vi "MAIN_test.vi"() -> ()   [LabVIEW 2023]
uses:
  <vilib>/Utility/file.llb/Write Delimited Spreadsheet (string).vi
  <vilib>/Utility/file.llb/Write Delimited Spreadsheet (I64).vi
  BT-Android_AE_library/BT-Android_interface.lvlib
  <resource>/objmgr/ni.dex.rc
panel:
  out "数组 4":i32[](array[numeric])
  out "数组 3":i32[](array[numeric])
  in  "?":enum32{"other test", "test 2"}(tab)
  out "End Character?":bool
  out "send timeout":bool=TRUE
  out "?":bool=TRUE
  in  "Send":bool
  in  "Data Send":string
  in  "Close Com":bool
  in  "timeout (10sec)":u32=10000
  out "status":bool
  out "code":i32
  out "source":string
  in  "temp varible":u16=4660 format="%x"
  out "single":u16(graph)
  in  "?":enum32{"初始化", "dynamic", "测试"}(tab)
  in  "local baud rate":u32=1000000
  in  "Select COM before run":refnum<visa-resource-name>="COM5"
  in  "Channels（包括检验）":i32=33
  in  "receive query frequency(ms)":i32=1
  in  "VISA size set":i32=10000
  in  "error queue size":i32=-1
  in  "receive file path (dialog if empty)":path=path "D:/Proj-labview/蓝牙无线采集/wireless-console/sd_data"
  in  "开始采集":bool
  in  "结束采集":bool
  out "data stream ele":i32
  out "VISA bytes now":i32
  in  "VISA bytes max":i32
  out "本次采样用时s":dbl format="%.2f"
  out "display array":u16[](array[numeric])
  out "接收字符串":string
  in  "采集选项":u16(ring) items=["上位机采集", "sd卡采集"]
  out "开始时间点":string="时间点字符串"
  in  "Receive":bool=TRUE
  out "data16 stream ele":i32
  in  "data16 save max":i32
  in  "data存盘":bool
  out "采样率PS":dbl format="%#_13g"
  out "Average Error Ratio":dbl format="%#.4f"
  in  "Right cycle":u64
  in  "Error cycle":i32
  in  "更新采样信息":bool=TRUE
  in  "error存盘":bool
  in  "mod":u8
  in  "清缓存":bool
  in  "data max ele":i32
  out "本次采样开始时间ms":u64
  in  "固定字符测试":bool
  out "时间打点":u64
  out "right cycle打点":u64
  out "35通道波形":u16[][](graph)
  # "通用设置："
  # "蓝牙设置："
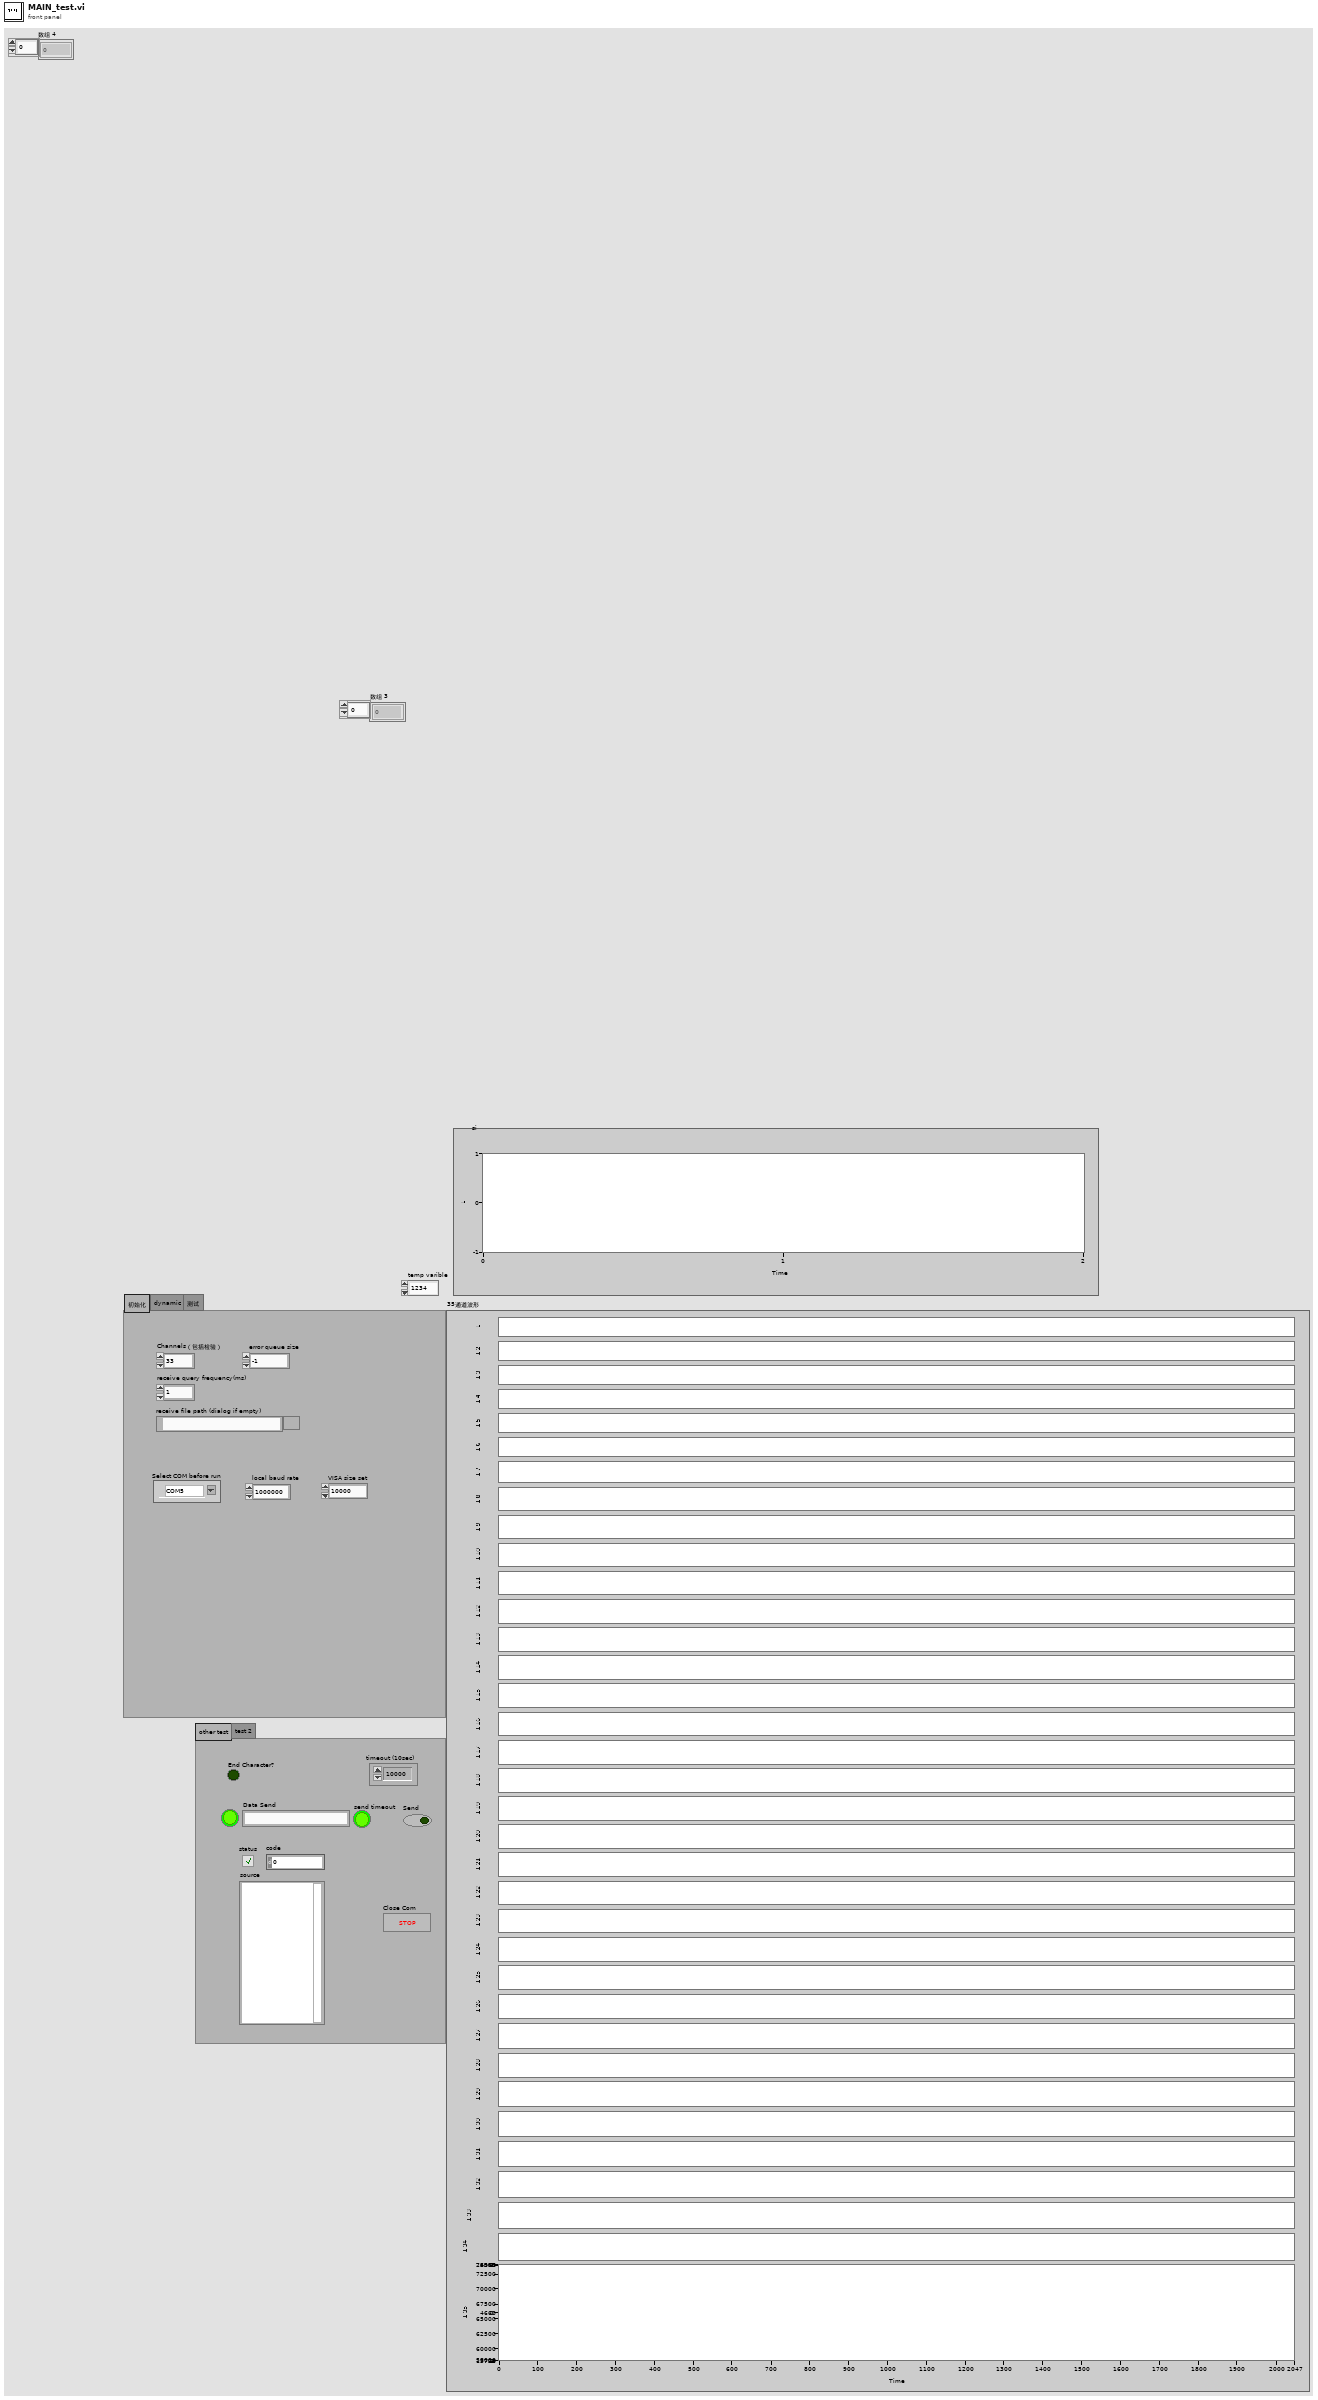
[diagram p1: front panel]
types:
  T1 = enum16{"init", "broadcast_data", "receive_data", "close", "clear_visa"}
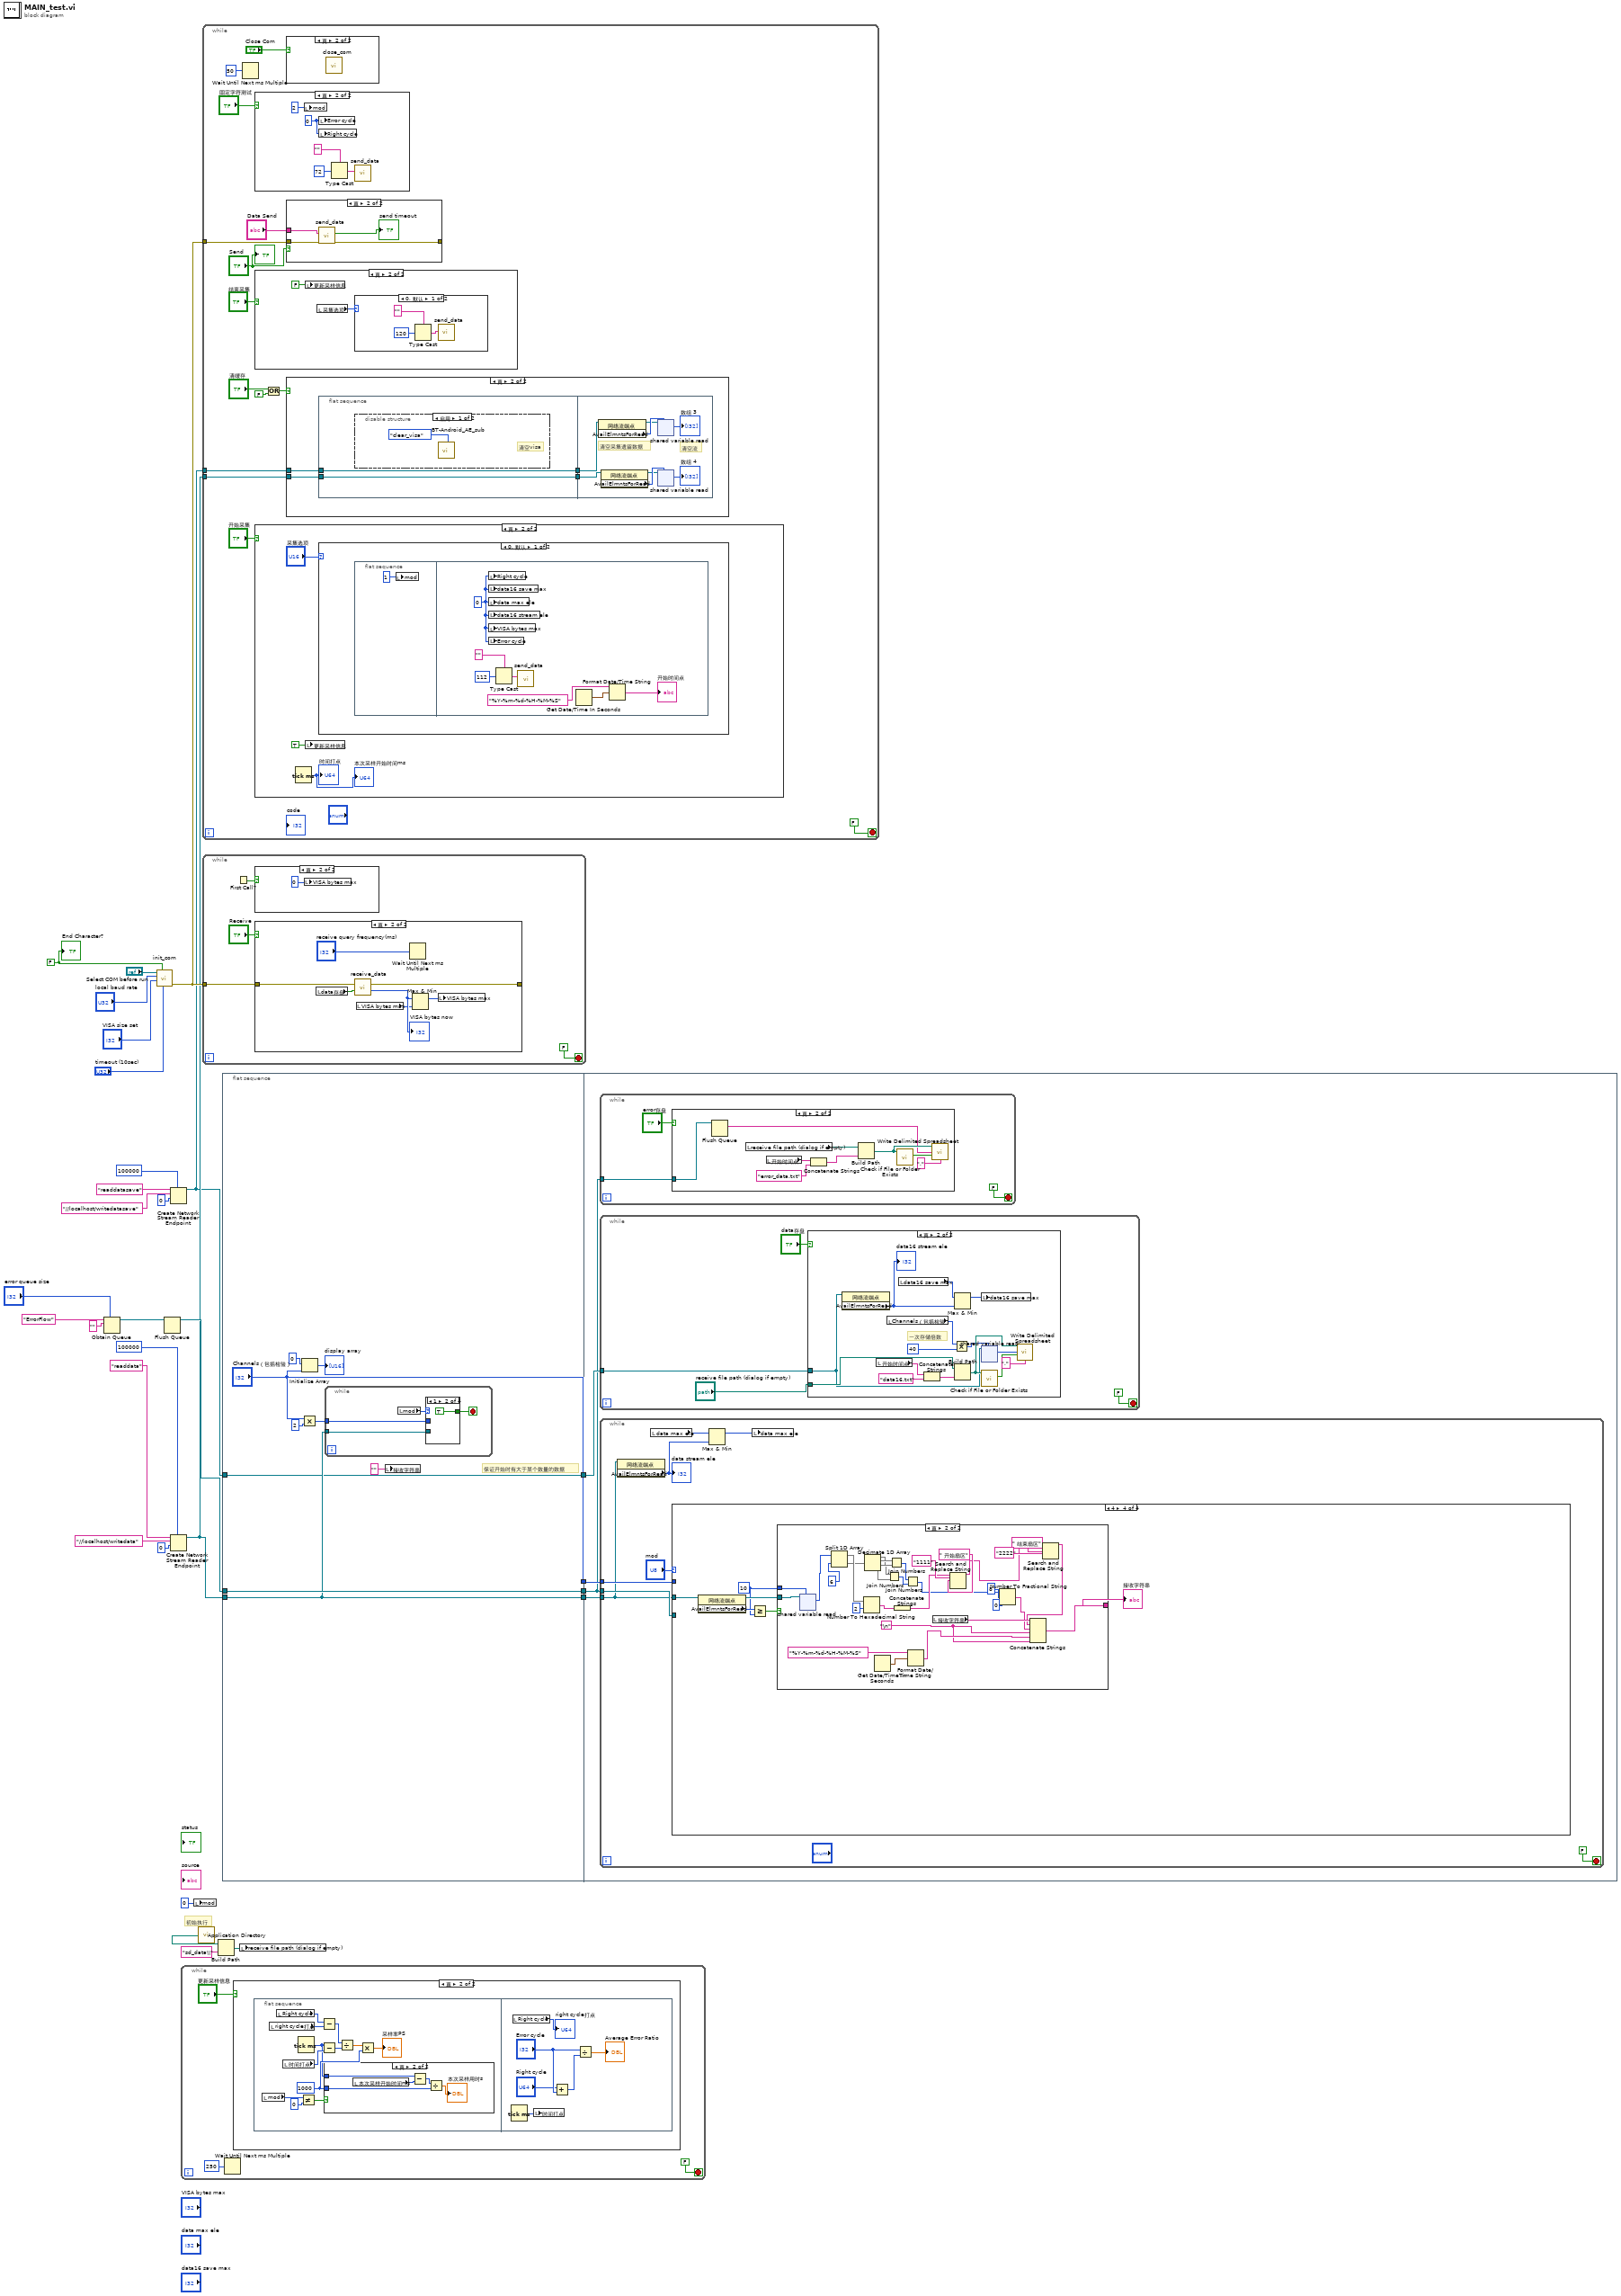
[diagram p0: block diagram]
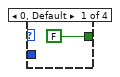
[diagram p4: hidden frame]
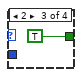
[diagram p5: hidden frame]
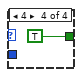
[diagram p6: hidden frame]
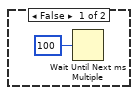
[diagram p7: hidden frame]
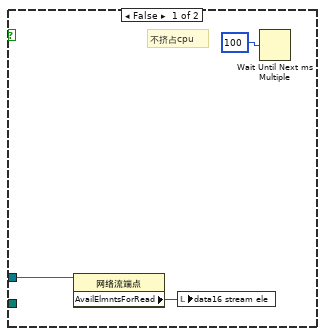
[diagram p8: hidden frame]
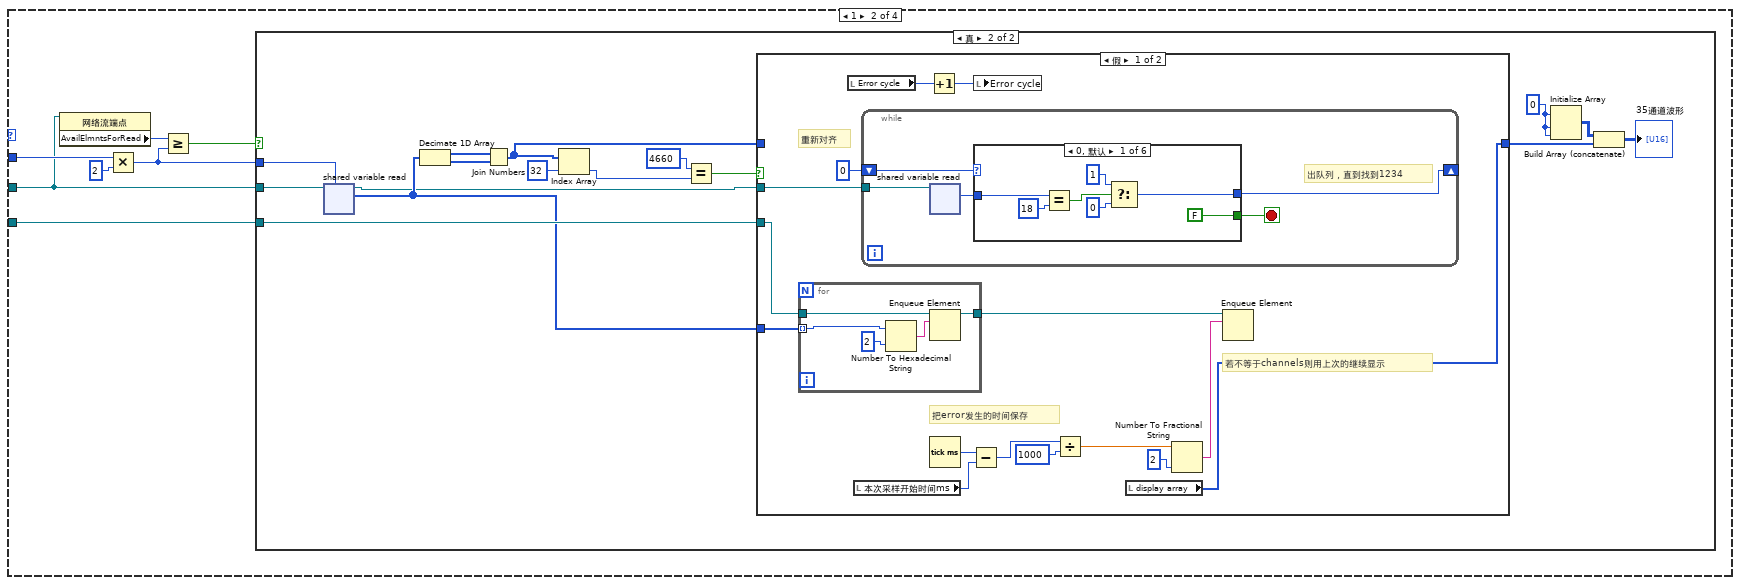
[diagram p10: hidden frame]
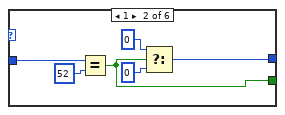
[diagram p12: hidden frame]
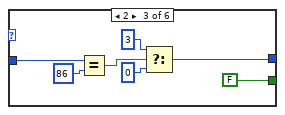
[diagram p13: hidden frame]
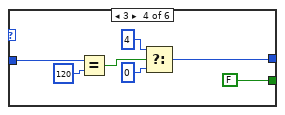
[diagram p14: hidden frame]
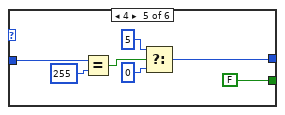
[diagram p15: hidden frame]
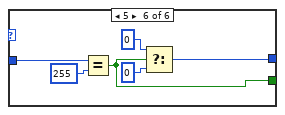
[diagram p16: hidden frame]
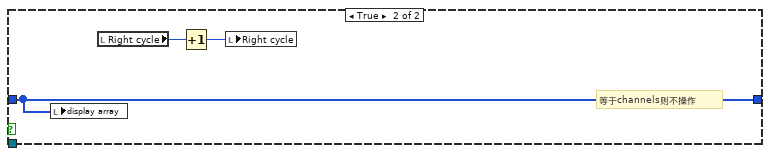
[diagram p17: hidden frame]
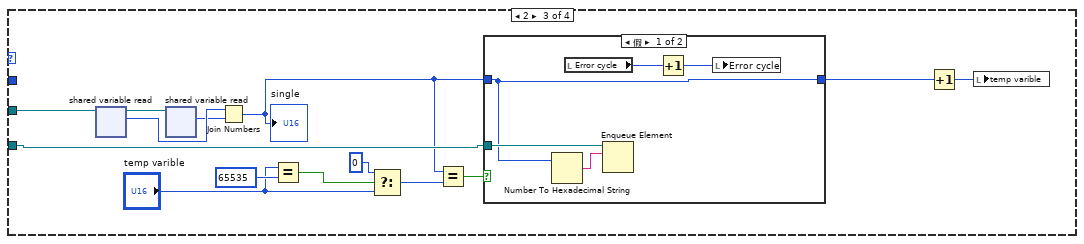
[diagram p18: hidden frame]
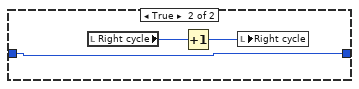
[diagram p19: hidden frame]
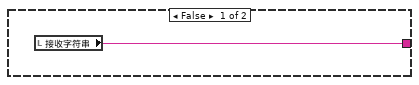
[diagram p20: hidden frame]
diagram:
  w26 = FALSE ("End Write on Termination Character?")
  # "初始执行"
  n1 = Obtain Queue(max queue size (-1, unlimited)="error queue size", name (unnamed)="ErrorFlow", element data type="") -> (queue out=w20:refnum<queue>)  [unwired: 2 in, 2 out]
  n2 = call "init_com.vi"("timeout (10sec)"="timeout (10sec)", "End Write on Termination Character?"=w26, "VISA buffer"="VISA size set", "baud rate"="local baud rate", "VISA resource name"="Select COM before run") -> ("error out"=w27:errorcluster)  [unwired: 6 in]
  n3 = Flush Queue(queue=w20) -> (queue out=w16:refnum<queue>)  [unwired: 1 in, 2 out]
  n4 = Create Network Stream Reader Endpoint(7:100000, 9:u16 0, 10:"//localhost/writedatasave", 11:"readdatasave") -> (3:w1:refnum<k21>)  [unwired: 3 in, 1 out]
  n5 = Create Network Stream Reader Endpoint(7:100000, 9:u8 0, 10:"//localhost/writedata", 11:"readdata") -> (3:w2:refnum<k21>)  [unwired: 3 in, 1 out]
  n6 = while {
    stop <- FALSE stop-if-true
    n7 = Wait Until Next ms Multiple(millisecond multiple=250) -> ()  [unwired: 1 out]
    n8 = case shown="真" "更新采样信息" {
      frame False {
      }
      frame True {
        n9 = flat-sequence {
          frame #0 {
            w34 = 1000
            n10 = local read "mod"() -> (w37:u8)
            n11 = local read "right cycle打点"() -> (w40:u64)
            n12 = local read "Right cycle"() -> (w38:u64)
            n13 = local read "时间打点"() -> (w41:u64)
            n14 = Tick Count (ms)() -> (millisecond timer value=w33:u32)
            n15 = Not Equal?(x=w37, y=0) -> (x != y?=w35:bool)
            n16 = Subtract(x=w38, y=w40) -> (x-y=w39:u64)
            n17 = Subtract(x=w33, y=w41) -> (x-y=w44:u64)
            n18 = case shown="真" w35 {
              tunnel: w34 -> [_ w47]
              tunnel: w33 -> [_ w46]
              frame False {
              }
              frame True {
                n19 = local read "本次采样开始时间ms"() -> (w45:u64)
                n20 = Subtract(x=w46, y=w45) -> (x-y=w48:u64)
                n21 = Divide(x=w48, y=w47) -> (x/y=→"本次采样用时s":dbl)
              }
            }
            n22 = Divide(x=w39, y=w44) -> (x/y=w42:dbl)
            n23 = Multiply(x=w42, y=w34) -> (x*y=→"采样率PS":dbl)
          }
          frame #1 {
            n24 = Tick Count (ms)() -> (millisecond timer value=w51:u32)
            n25 = local read "Right cycle"() -> (→"right cycle打点":u64)
            n26 = local write "时间打点"(w51) -> ()
            n27 = Add(x="Right cycle", y="Error cycle") -> (x+y=w54:u64)
            n28 = Divide(x="Error cycle", y=w54) -> (x/y=→"Average Error Ratio":dbl)
          }
        }
      }
    }
  }
  n29 = local write "mod"(0) -> ()
  n30 = call <vilib>:"Application Directory.vi"() -> ("Application Directory"=w14:path)
  n31 = while {
    tunnel: w27 -> [w68]
    tunnel: w2 -> [w61]
    tunnel: w1 -> [w60]
    stop <- FALSE ("End Write on Termination Character?") stop-if-true
    n32 = Wait Until Next ms Multiple(millisecond multiple=50) -> ()  [unwired: 1 out]
    n33 = case shown="真" "固定字符测试" {
      frame False {
      }
      frame True {
        w85 = 0
        n34 = local write "mod"(2) -> ()
        n35 = local write "Error cycle"(w85) -> ()
        n36 = local write "Right cycle"(w85) -> ()
        n37 = Type Cast(type="" ("Data Send 2"), x=72) -> (*(type *) &x=w87:string)
        n38 = call "send_data.vi"("send data (string)"=w87) -> ()  [unwired: 9 in, 2 out]
      }
    }
    n39 = case shown="真" "结束采集" {
      frame False {
      }
      frame True {
        n40 = local write "更新采样信息"(FALSE) -> ()
        n41 = local read "采集选项"() -> (w91:u16)
        n42 = case shown="0, 默认" w91 {
          frame 0, Default {
            n43 = Type Cast(type="" ("Data Send 2"), x=120) -> (*(type *) &x=w94:string)
            n44 = call "send_data.vi"("send data (string)"=w94) -> ()  [unwired: 9 in, 2 out]
          }
          frame 1 {
            n45 = Type Cast(type="" ("Data Send 2"), x=114) -> (*(type *) &x=w95:string)
            n46 = call "send_data.vi"("send data (string)"=w95) -> ()  [unwired: 9 in, 2 out]
          }
        }
      }
    }
    n47 = case shown="真" "开始采集" {
      frame False {
      }
      frame True {
        n48 = Tick Count (ms)() -> (millisecond timer value=→"本次采样开始时间ms" →"时间打点":u32)
        n49 = local write "更新采样信息"(TRUE) -> ()
        n50 = case shown="0, 默认" "采集选项" {
          frame 0, Default {
            n51 = flat-sequence {
              frame #0 {
                n52 = local write "mod"(1) -> ()
              }
              frame #1 {
                w107 = 0
                n53 = local write "Right cycle"(w107) -> ()
                n54 = local write "data16 save max"(w107) -> ()
                n55 = local write "data max ele"(w107) -> ()
                n56 = local write "data16 stream ele"(w107) -> ()
                n57 = local write "VISA bytes max"(w107) -> ()
                n58 = local write "Error cycle"(w107) -> ()
                n59 = Type Cast(type="" ("Data Send 2"), x=112) -> (*(type *) &x=w108:string)
                n60 = call "send_data.vi"("send data (string)"=w108) -> ()  [unwired: 9 in, 2 out]
                n61 = Get Date/Time In Seconds() -> (seconds since 1Jan1904=w104:timestamp)
                n62 = Format Date/Time String(time format string (%c)="%Y-%m-%d-%H-%M-%S", seconds (now)=w104) -> (date/time string=→"开始时间点":string)  [unwired: 1 in]
              }
            }
          }
          frame 1 {
            n63 = flat-sequence {
              frame #0 {
                n64 = local write "mod"(4) -> ()
              }
              frame #1 {
                w110 = FALSE
                # "sd采集"
                n65 = local write "data存盘"(w110) -> ()
                n66 = local write "error存盘"(w110) -> ()
                n67 = Type Cast(type="" ("Data Send 2"), x=115) -> (*(type *) &x=w116:string)
                n68 = call "send_data.vi"("send data (string)"=w116) -> ()  [unwired: 9 in, 2 out]
                n69 = Get Date/Time In Seconds() -> (seconds since 1Jan1904=w113:timestamp)
                n70 = Format Date/Time String(time format string (%c)="%Y-%m-%d-%H-%M-%S", seconds (now)=w113) -> (date/time string=w111:string)  [unwired: 1 in]
                n71 = local write "开始时间点"(w111) -> ()
              }
            }
          }
        }
      }
    }
    n72 = Or(x="清缓存", y=FALSE) -> (x .or. y?=w57:bool)
    n73 = case shown="真" "Close Com" {
      frame False {
      }
      frame True {
        n74 = call "close_com.vi"() -> ()  [unwired: 11 in, 1 out]
      }
    }
    n75 = case shown="真" "Send" {
      tunnel: "Data Send" -> [_ w121]
      tunnel: w68 -> [w117 w120]
      tunnel: [w117 w119] -> _
      frame False {
      }
      frame True {
        n76 = call "send_data.vi"("error in (no error)"=w120, "send data (string)"=w121) -> ("error out"=w119:errorcluster, "timeout?"=→"send timeout":bool)  [unwired: 8 in]
      }
    }
    n77 = case shown="真" w57 {
      tunnel: w61 -> [_ w71]
      tunnel: w60 -> [_ w70]
      frame False {
      }
      frame True {
        n78 = flat-sequence {
          tunnel: w70 -> [w74]
          tunnel: w71 -> [w75]
          tunnel: [w75] -> w73
          tunnel: [w74] -> w72
          tunnel: w73 -> [w80]
          tunnel: w72 -> [w79]
          frame #0 {
            n79 = disable-structure shown="启用" {
              frame Enabled {
                # "清空visa"
                n80 = call "BT-Android_AE_sub.vi"("mode"=T1."clear_visa") -> ()  [unwired: 16 in, 3 out]
              }
              frame Disabled {
              }
            }
          }
          frame #1 {
            # "清空采集遗留数据"
            # "清空流"
            n81 = property on="属性节点" class="网络流端点"(reference=w79) -> (reference out=w82:refnum<k21>, "AvailElmntsForRead"=w84:i32)  [unwired: 1 in, 1 out]
            n82 = property on="属性节点" class="网络流端点"(reference=w80) -> (reference out=w81:refnum<k21>, "AvailElmntsForRead"=w83:i32)  [unwired: 1 in, 1 out]
            n83 = shared-variable-read(w82, w84) -> (→"数组 3":u16[])  [unwired: 2 in, 3 out]
            n84 = shared-variable-read(w81, w83) -> (→"数组 4":u8[])  [unwired: 2 in, 3 out]
          }
        }
      }
    }
    "?" <- "Send"
  }
  n85 = while {
    tunnel: w27 -> [w124]
    stop <- FALSE ("End Write on Termination Character?") stop-if-true
    n86 = First Call?() -> (First Call?: T/F=w122:bool)
    n87 = case shown="真" w122 {
      frame False {
      }
      frame True {
        n88 = local write "VISA bytes max"(0) -> ()
      }
    }
    n89 = case shown="真" "Receive" {
      tunnel: w124 -> [w127 w134]
      tunnel: [w127 w133] -> _
      frame False {
      }
      frame True {
        n90 = local read "data存盘"() -> (w129:bool)
        n91 = call "receive_data.vi"("error in (no error)"=w134, "data保存"=w129) -> ("error out"=w133:errorcluster, "VISA bytes now"=w131:i32)  [unwired: 11 in, 1 out]
        "VISA bytes now" <- w131
        n92 = local read "VISA bytes max"() -> (w130:i32)
        n93 = Wait Until Next ms Multiple(millisecond multiple="receive query frequency(ms)") -> ()  [unwired: 1 out]
        n94 = Max & Min(x=w131, y=w130) -> (max(x,y)=w128:i32)  [unwired: 1 out]
        n95 = local write "VISA bytes max"(w128) -> ()
      }
    }
  }
  n96 = Build Path(base path=w14, name or relative path="sd_data\\") -> (appended path=w12:path)
  n97 = flat-sequence {
    tunnel: [w136] -> w24
    tunnel: ["Channels（包括检验）"] -> w23
    tunnel: [w135] -> w21
    tunnel: [w141] -> w17
    tunnel: w16 -> [w141]
    tunnel: w2 -> [w136]
    tunnel: w1 -> [w135]
    tunnel: w24 -> [w155]
    tunnel: w23 -> [w154]
    tunnel: w21 -> [w153]
    tunnel: w17 -> [w152]
    frame #0 {
      # "保证开始时有大于某个数量的数据"
      n98 = Multiply(x="Channels（包括检验）", y=2) -> (x*y=w138:i32)
      n99 = Initialize Array(u16 0, "Channels（包括检验）") -> (→"display array":u16[])
      n100 = while {
        tunnel: w138 -> [w147]
        tunnel: w136 -> [w144]
        stop <- w146 stop-if-true
        n101 = local read "mod"() -> (w145:u8)
        n102 = case shown="1" w145 {
          tunnel: w147 -> [_ _ _ _]
          tunnel: [FALSE TRUE TRUE TRUE] -> w146
          tunnel: w144 -> [_ _ _ _]
          frame 0, Default {
          }
          frame 1 {
          }
          frame 2 {
          }
          frame 4 {
          }
        }
      }
      n103 = local write "接收字符串"("") -> ()
    }
    frame #1 {
      n104 = while {
        tunnel: w152 -> [w156]
        stop <- FALSE stop-if-true
        n105 = case shown="真" "error存盘" {
          tunnel: w156 -> [_ w164]
          frame False {
            n106 = Wait Until Next ms Multiple(millisecond multiple=100) -> ()  [unwired: 1 out]
          }
          frame True {
            n107 = Flush Queue(queue=w164) -> (remaining elements=w163:string[])  [unwired: 1 in, 2 out]
            n108 = local read "receive file path (dialog if empty)"() -> (w165:path)
            n109 = local read "开始时间点"() -> (w162:string)
            n110 = Concatenate Strings(w162, "error_data.txt" ("name or relative path")) -> (w160:string)
            n111 = Build Path(base path=w165, name or relative path=w160) -> (appended path=w168:path)
            n112 = call <vilib>:"Check if File or Folder Exists.vi"("path"=w168) -> ("file or folder exists?"=w167:bool)  [unwired: 8 in, 2 out]
            n113 = call-poly <vilib>:"Write Delimited Spreadsheet.vi"("file path (dialog if empty)"=w168, "1D data"=w163, "append to file? (new file:F)"=w167, "delimiter (\\t)"="," ("delimiter (\\t)")) -> ()  [unwired: 10 in, 2 out]
          }
        }
      }
      n114 = while {
        tunnel: w153 -> [w169]
        stop <- FALSE stop-if-true
        n115 = case shown="真" "data存盘" {
          tunnel: "receive file path (dialog if empty)" -> [_ w188]
          tunnel: w169 -> [w174 w181]
          frame False {
            # "不挤占cpu"
            n116 = property on="属性节点" class="网络流端点"(reference=w174) -> ("AvailElmntsForRead"=w173:i32)  [unwired: 1 in, 2 out]
            n117 = local write "data16 stream ele"(w173) -> ()
            n118 = Wait Until Next ms Multiple(millisecond multiple=100) -> ()  [unwired: 1 out]
          }
          frame True {
            # "一次存储倍数"
            n119 = property on="属性节点" class="网络流端点"(reference=w181) -> ("AvailElmntsForRead"=w180:i32)  [unwired: 1 in, 2 out]
            "data16 stream ele" <- w180
            n120 = local read "开始时间点"() -> (w179:string)
            n121 = local read "Channels（包括检验）"() -> (w185:i32)
            n122 = local read "data16 save max"() -> (w186:i32)
            n123 = Concatenate Strings(w179, "data16.txt" ("name or relative path")) -> (w177:string)
            n124 = Multiply(x=w185, y=40) -> (x*y=w183:i32)
            n125 = Max & Min(x=w186, y=w180) -> (max(x,y)=w176:i32)  [unwired: 1 out]
            n126 = Build Path(base path=w188, name or relative path=w177) -> (appended path=w189:path)
            n127 = local write "data16 save max"(w176) -> ()
            n128 = shared-variable-read(w181, w183) -> (w182:u16[])  [unwired: 2 in, 3 out]
            n129 = call <vilib>:"Check if File or Folder Exists.vi"("path"=w189) -> ("file or folder exists?"=w190:bool)  [unwired: 8 in, 2 out]
            n130 = call-poly <vilib>:"Write Delimited Spreadsheet.vi"("file path (dialog if empty)"=w189, "1D data"=w182, "append to file? (new file:F)"=w190, "delimiter (\\t)"=",") -> ()  [unwired: 10 in, 2 out]
          }
        }
      }
      n131 = while {
        tunnel: w154 -> [w197]
        tunnel: w155 -> [w193]
        tunnel: w152 -> [w194]
        stop <- FALSE ("End Write on Termination Character?") stop-if-true
        n132 = property on="属性节点" class="网络流端点"(reference=w193) -> ("AvailElmntsForRead"=w192:i32)  [unwired: 1 in, 2 out]
        "data stream ele" <- w192
        n133 = local read "data max ele"() -> (w195:i32)
        n134 = case shown="4" "mod" {
          tunnel: w197 -> [_ w203 _ _]
          tunnel: w193 -> [_ w202 w293 w315]
          tunnel: w194 -> [_ w205 w302 _]
          frame 0, Default {
          }
          frame 1 {
            n135 = property on="属性节点" class="网络流端点"(reference=w202) -> ("AvailElmntsForRead"=w201:i32)  [unwired: 1 in, 2 out]
            n136 = Multiply(x=w203, y=2) -> (x*y=w200:i32)
            n137 = Greater Or Equal?(x=w201, y=w200) -> (x >= y?=w199:bool)
            n138 = case shown="真" w199 {
              tunnel: w205 -> [_ w213]
              tunnel: w202 -> [_ w209]
              tunnel: w200 -> [_ w206]
              frame False {
              }
              frame True {
                w217 = u16 0
                n139 = shared-variable-read(w209, w206) -> (w207:refnum<k21>, w208:u8[])  [unwired: 2 in, 2 out]
                n140 = Decimate 1D Array(w208) -> (w221:u8[], w220:u8[])
                n141 = Join Numbers(hi=w221, lo=w220) -> ((hi.lo)=w211:u16[])
                n142 = Index Array(array=w211, index=32) -> (element=w215:u16)
                n143 = Equal?(x=u16 4660, y=w215) -> (x = y?=w210:bool)
                n144 = case shown="假" w210 {
                  tunnel: [w236 w289] -> w214
                  tunnel: w211 -> [_ w289]
                  tunnel: w213 -> [w235 _]
                  tunnel: w208 -> [w234 _]
                  tunnel: w207 -> [w223 _]
                  frame False {
                    # "把error发生的时间保存"
                    # "重新对齐"
                    # "若不等于channels则用上次的继续显示"
                    n145 = for {
                      tunnel: w234 -> [w285] mode=indexing
                      tunnel: w235 -> [w286]
                      tunnel: [w282] -> w225
                      n146 = Number To Hexadecimal String(1:2, 2:w285) -> (0:w283:string)
                      n147 = Enqueue Element(queue=w286, element=w283) -> (queue out=w282:refnum<queue>)  [unwired: 2 in, 2 out]
                    }
                    n148 = local read "Error cycle"() -> (w233:i32)
                    n149 = local read "本次采样开始时间ms"() -> (w230:u64)
                    n150 = while {
                      shift-right: [w240] -> _
                      shift-left: 0 -> [w241]
                      tunnel: w223 -> [w237]
                      stop <- w239 stop-if-true
                      # "出队列，直到找到1234"
                      n151 = shared-variable-read(w237) -> (w238:u8)  [unwired: 2 in, 3 out]
                      n152 = case shown="0, 默认" w241 {
                        tunnel: [w243 w251 w258 w265 w269 w277] -> w240
                        tunnel: w238 -> [w246 w252 w259 w266 w271 w278]
                        tunnel: [FALSE w249 FALSE FALSE FALSE w276] -> w239
                        frame 0, Default {
                          n153 = Equal?(x=w246, y=18) -> (x = y?=w247:bool)
                          n154 = Select(t=1, s=w247, f=0) -> (s? t:f=w243:i32)
                        }
                        frame 1 {
                          n155 = Equal?(x=w252, y=52) -> (x = y?=w249:bool)
                          n156 = Select(t=0, s=w249, f=0) -> (s? t:f=w251:i32)
                        }
                        frame 2 {
                          n157 = Equal?(x=w259, y=86) -> (x = y?=w257:bool)
                          n158 = Select(t=3, s=w257, f=0) -> (s? t:f=w258:i32)
                        }
                        frame 3 {
                          n159 = Equal?(x=w266, y=120) -> (x = y?=w263:bool)
                          n160 = Select(t=4, s=w263, f=0) -> (s? t:f=w265:i32)
                        }
                        frame 4 {
                          n161 = Equal?(x=w271, y=255) -> (x = y?=w272:bool)
                          n162 = Select(t=5, s=w272, f=0) -> (s? t:f=w269:i32)
                        }
                        frame 5 {
                          n163 = Equal?(x=w278, y=255) -> (x = y?=w276:bool)
                          n164 = Select(t=0, s=w276, f=0) -> (s? t:f=w277:i32)
                        }
                      }
                    }
                    n165 = Increment(x=w233) -> (x+1=w232:i32)
                    n166 = Tick Count (ms)() -> (millisecond timer value=w231:u32)
                    n167 = Subtract(x=w231, y=w230) -> (x-y=w229:u64)
                    n168 = local write "Error cycle"(w232) -> ()
                    n169 = Divide(x=w229, y=1000) -> (x/y=w227:dbl)
                    n170 = local read "display array"() -> (w236:u16[])
                    n171 = Number To Fractional String(number=w227, precision (6)=2) -> (F-format string=w224:string)  [unwired: 2 in]
                    n172 = Enqueue Element(queue=w225, element=w224) -> ()  [unwired: 2 in, 3 out]
                  }
                  frame True {
                    # "等于channels则不操作"
                    n173 = local write "display array"(w289) -> ()
                    n174 = local read "Right cycle"() -> (w288:u64)
                    n175 = Increment(x=w288) -> (x+1=w287:u64)
                    n176 = local write "Right cycle"(w287) -> ()
                  }
                }
                n177 = Initialize Array(w217, w217, w217) -> (w218:u16[][])
                n178 = Build Array (concatenate)(w218, w214) -> (→"35通道波形":u16[][])
              }
            }
          }
          frame 2 {
            n179 = shared-variable-read(w293) -> (w292:refnum<k21>, w291:u8)  [unwired: 2 in, 2 out]
            n180 = shared-variable-read(w292) -> (w290:u8)  [unwired: 2 in, 3 out]
            n181 = Join Numbers(hi=w291, lo=w290) -> ((hi.lo)=w297:u16)
            "single" <- w297
            n182 = Equal?(x="temp varible", y=65535) -> (x = y?=w300:bool)
            n183 = Select(t=0, s=w300, f="temp varible") -> (s? t:f=w298:i32)
            n184 = Equal?(x=w297, y=w298) -> (x = y?=w303:bool)
            n185 = case shown="假" w303 {
              tunnel: w297 -> [w305 w309]
              tunnel: w302 -> [w306 _]
              tunnel: [w305 w309] -> w295
              frame False {
                n186 = Number To Hexadecimal String(2:w305) -> (0:w304:string)  [unwired: 1 in]
                n187 = local read "Error cycle"() -> (w308:i32)
                n188 = Enqueue Element(queue=w306, element=w304) -> ()  [unwired: 2 in, 3 out]
                n189 = Increment(x=w308) -> (x+1=w307:i32)
                n190 = local write "Error cycle"(w307) -> ()
              }
              frame True {
                n191 = local read "Right cycle"() -> (w311:u64)
                n192 = Increment(x=w311) -> (x+1=w310:u64)
                n193 = local write "Right cycle"(w310) -> ()
              }
            }
            n194 = Increment(x=w295) -> (x+1=w294:u16)
            n195 = local write "temp varible"(w294) -> ()
          }
          frame 4 {
            w312 = 10
            n196 = property on="属性节点" class="网络流端点"(reference=w315) -> (reference out=w313:refnum<k21>, "AvailElmntsForRead"=w314:i32)  [unwired: 1 in, 1 out]
            n197 = Greater Or Equal?(x=w314, y=w312) -> (x >= y?=w317:bool)
            n198 = case shown="真" w317 {
              tunnel: [w318 w320] -> w316
              tunnel: w313 -> [_ w347]
              tunnel: w312 -> [_ w346]
              frame False {
                n199 = local read "接收字符串"() -> (w318:string)
              }
              frame True {
                w321 = "\n"
                n200 = shared-variable-read(w347, w346) -> (w338:u8[])  [unwired: 2 in, 3 out]
                n201 = Split 1D Array(array=w338, index=6) -> (first subarray=w336:u8[], second subarray=w325:u8[])
                n202 = Number To Hexadecimal String(1:2, 2:w336) -> (0:w335:string[])
                n203 = Decimate 1D Array(w325) -> (w333:u8[], w332:u8[], w331:u8[], w330:u8[])
                n204 = Get Date/Time In Seconds() -> (seconds since 1Jan1904=w345:timestamp)
                n205 = Join Numbers(hi=w331, lo=w330) -> ((hi.lo)=w328:u16[])
                n206 = Join Numbers(hi=w333, lo=w332) -> ((hi.lo)=w329:u16[])
                n207 = Concatenate Strings(w335) -> (w334:string)
                n208 = Join Numbers(hi=w329, lo=w328) -> ((hi.lo)=w324:u32[])
                n209 = Format Date/Time String(time format string (%c)="%Y-%m-%d-%H-%M-%S", seconds (now)=w345) -> (date/time string=w322:string)  [unwired: 1 in]
                n210 = local read "接收字符串"() -> (w348:string)
                n211 = Search and Replace String(input string=w334, search string="1111", replace string=" 开始扇区") -> (result string=w339:string)  [unwired: 5 in, 3 out]
                n212 = Number To Fractional String(number=w324, width (-)=8, precision (6)=0) -> (F-format string=w319:string[])  [unwired: 1 in]
                n213 = Search and Replace String(input string=w339, search string="2222", replace string=" 结束扇区") -> (result string=w323:string)  [unwired: 5 in, 3 out]
                n214 = Concatenate Strings(w348, w323, w319, w321, w322, w321) -> (w320:string)
              }
            }
            "接收字符串" <- w316
          }
        }
        n215 = Max & Min(x=w195, y=w192) -> (max(x,y)=w191:i32)  [unwired: 1 out]
        n216 = local write "data max ele"(w191) -> ()
      }
    }
  }
  n217 = local write "receive file path (dialog if empty)"(w12) -> ()
  "End Character?" <- w26
